vi "Store New Token.vi"(7 "Config File Name":string="config.ini", 8 "error in (no error)":errorcluster, 11 "token response (JSON)":string) -> (0 "error out":errorcluster)   [LabVIEW 2020, in "Netatmo-WeatherStation.lvlib"]
uses:
  Netatmo-WeatherStation.lvlib
  38c82571-bc5e-46af-bf68-39e55817eb04.vi
  452556e5-531e-4f67-82e4-728213015fb2.vi
  ca94afaa-7ef3-4ada-bc32-b76fa4498785.vi
  <vilib>/JDP Science/JSONtext/Find Item.vi
  <vilib>/JDP Science/JSONtext/String Subset.vi
  <vilib>/JDP Science/JSONtext/Parsing/Parse Full Path or Item Name.vi
  <vilib>/JDP Science/JSONtext/Next JSON Value.vi
  <vilib>/JDP Science/JSONtext/support/Error Cluster From Code.vi
  <vilib>/JDP Science/JSONtext/Offset/Find Item Locations by Path.vi
  <vilib>/JDP Science/JSONtext/JSON text to Variant.vi
  globals.vi
  <vilib>/Utility/config.llb/NI_LVConfig.lvlib
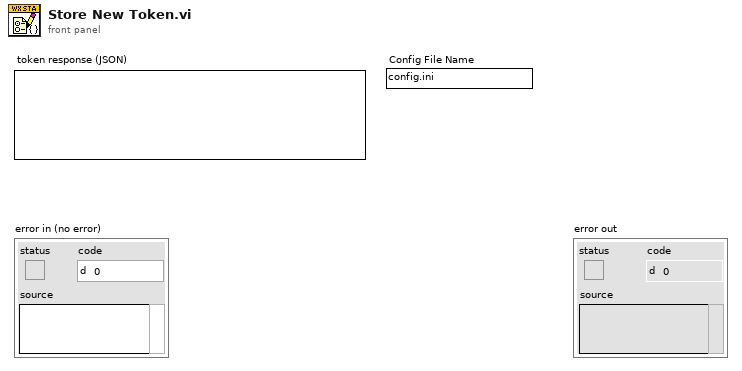
[diagram p1: front panel]
types:
  T1 = cluster{"access_token":string, "refresh_token":string, "expire_time":timestamp}
  T2 = typedef "NI_LVConfig.lvlib/Config Data RefNum.ctl" = refnum<k1>
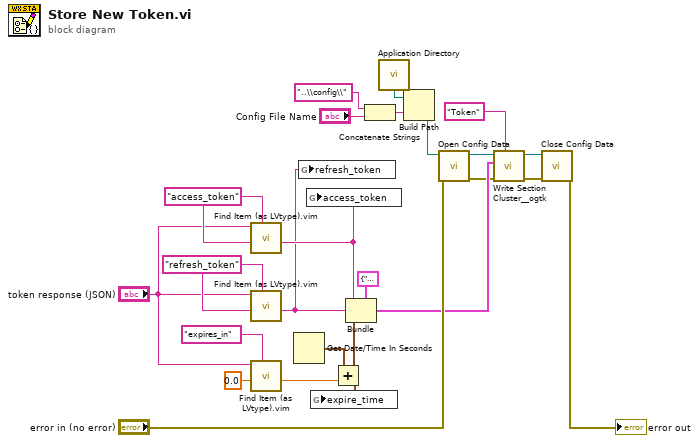
[diagram p0: block diagram]
diagram:
  w12 = "refresh_token" ("$Path or Item Name")
  w13 = "access_token" ("$Path or Item Name")
  n1 = call "Find Item (as LVtype).vim"("$Path or Item Name"=w13, "Data Type and Default Value"=w13, "JSON"="token response (JSON)") -> ("Data"=w3:string)  [unwired: 5 in, 3 out]
  n2 = call "Find Item (as LVtype).vim"("$Path or Item Name"=w12, "Data Type and Default Value"=w12, "JSON"="token response (JSON)") -> ("Data"=w2:string)  [unwired: 5 in, 3 out]
  n3 = call "Find Item (as LVtype).vim"("$Path or Item Name"="expires_in", "Data Type and Default Value"=0.0, "JSON"="token response (JSON)") -> ("Data"=w8:dbl)  [unwired: 5 in, 3 out]
  n4 = Get Date/Time In Seconds() -> (seconds since 1Jan1904=w19:timestamp)
  n5 = global write "globals.vi" "refresh_token"(w2) -> ()
  n6 = global write "globals.vi" "access_token"(w3) -> ()
  n7 = Add(x=w19, y=w8) -> (x+y=w1:timestamp)
  n8 = global write "globals.vi" "expire_time"(w1) -> ()
  n9 = Bundle(cluster=T1 {"access_token"="", "refresh_token"="", "expire_time"=timestamp(0 s since 1904-01-01)}, "access_token"=w3, "refresh_token"=w2, "expire_time"=w1) -> (w17:T1)
  n10 = Concatenate Strings("..\\config\\" ("format string"), "Config File Name") -> (w4:string)
  n11 = call <vilib>:"Application Directory.vi"() -> ("Application Directory"=w24:path)
  n12 = Build Path(base path=w24, name or relative path=w4) -> (appended path=w23:path)
  n13 = call <vilib>:"Open Config Data.vi"("error in (no error)"="error in (no error)", "configuration file path"=w23) -> ("error out"=w16:errorcluster, "refnum"=w21:T2)  [unwired: 7 in, 1 out]
  n14 = call <userlib>:"Write Section Cluster__ogtk.vi"("section (optional)"="Token", "error in (no error)"=w16, "Section Formatted Cluster"=w17, "refnum"=w21) -> ("error out"=w15:errorcluster, "dup refnum"=w18:T2)  [unwired: 6 in]
  n15 = call <vilib>:"Close Config Data.vi"("error in (no error)"=w15, "refnum"=w18) -> ("error out"=→"error out":errorcluster)  [unwired: 8 in, 1 out]
